vi "Configure Output Channel Coupling.vi"(8 "error in (no error)":errorcluster, 10 "Coupling Channel (0: None)":i32(ring) items=["None", "All", "Channel 1 And 2", "Channel 1 And 3", "Channel 2 And 3"], 11 "VISA resource name":refnum<visa-resource-name>) -> (0 "error out":errorcluster, 3 "VISA resource name out":refnum<visa-resource-name>)   [LabVIEW 2020, in "Keysight E36300 Series.lvlib"]
doc: "Configures the output channels are controlled by the output synchronization function.\n\n<b>Notes:</b>\n(1)This VI is not applicable for EDU36311A model.\n(2)This VI sets output channels to the OFF state. \n(3)<b>Reset</b> VI doesn't affect the coupling of the output channel."
uses:
  Keysight E36300 Series.lvlib
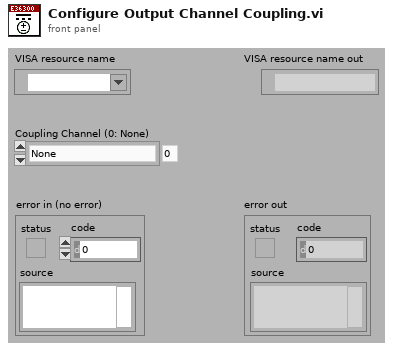
[diagram p1: front panel]
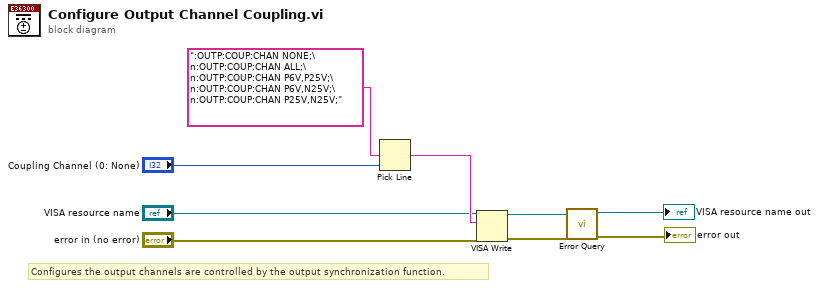
[diagram p0: block diagram]
diagram:
  # "Configures the output channels are controlled by the output synchronization function."
  n1 = Pick Line(multi-line string=":OUTP:COUP:CHAN NONE;\n:OUTP:COUP:CHAN ALL;\n:OUTP:COUP:CHAN P6V,P25V;\n:OUTP:COUP:CHAN P6V,N25V;\n:OUTP:COUP:CHAN P25V,N25V;", line index="Coupling Channel (0: None)") -> (output string=w6:string)  [unwired: 1 in]
  n2 = VISA Write(VISA resource name="VISA resource name", write buffer=w6, error in (no error)="error in (no error)") -> (VISA resource name out=w5:refnum<visa-resource-name>, error out=w2:errorcluster)  [unwired: 1 out]
  n3 = call "Error Query.vi"("error in (no error)"=w2, "VISA resource name"=w5) -> ("error out"=→"error out":errorcluster, "VISA resource name out"=→"VISA resource name out":refnum<visa-resource-name>)  [unwired: 6 in, 2 out]
